vi "InstaCoverage Time Measurement - Copy.vi"(10 "test file paths":path[](array[path]), 11 "All Test":bool=TRUE) -> (2 "ICov Results":enum16{"PASSED", "FAILED", "ERROR"}[](array[ring]), 3 "ICov Testing time (seconds)":dbl)   [LabVIEW 2018]
uses:
  <vilib>/InstaCoverage/Pro/InstaCoverage_API/Run Tests From Project By Path.vi
  <vilib>/InstaCoverage/Core/TestSuite/TestSuite.lvclass
  <vilib>/InstaCoverage/Pro/InstaCoveragePro.lvlib
panel:
  out "Project Path":string
  # "If \"All Test\" is true, then all tests will be executed independelntly \nof \"test file paths\"."
  # "ICov"
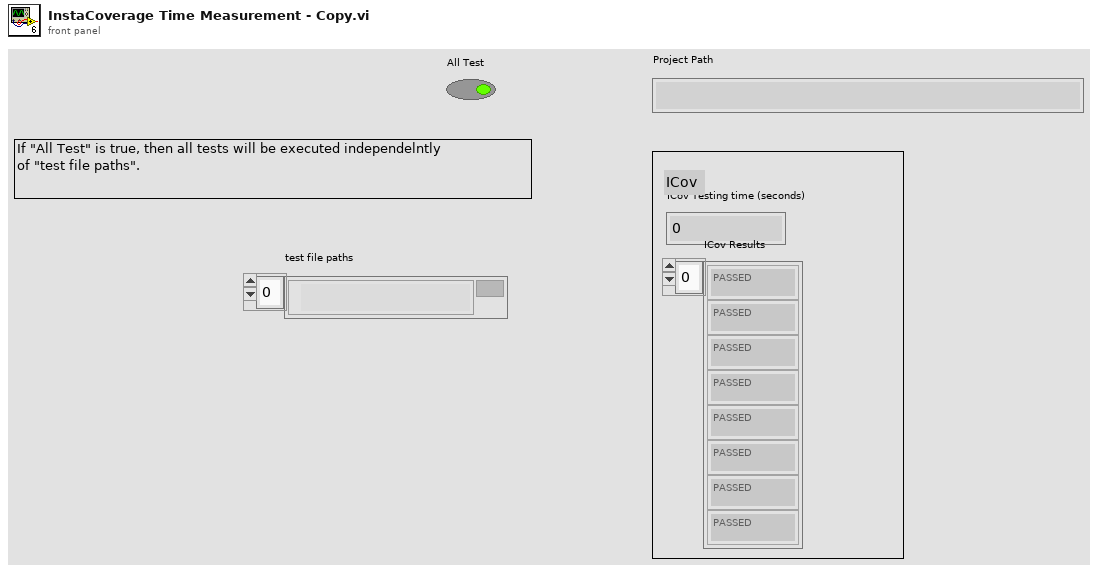
[diagram p1: front panel]
types:
  T1 = typedef "InstaCoverageCore.lvlib/APIResultEnum.ctl" = enum16{"PASSED", "FAILED", "ERROR", "NONE"}
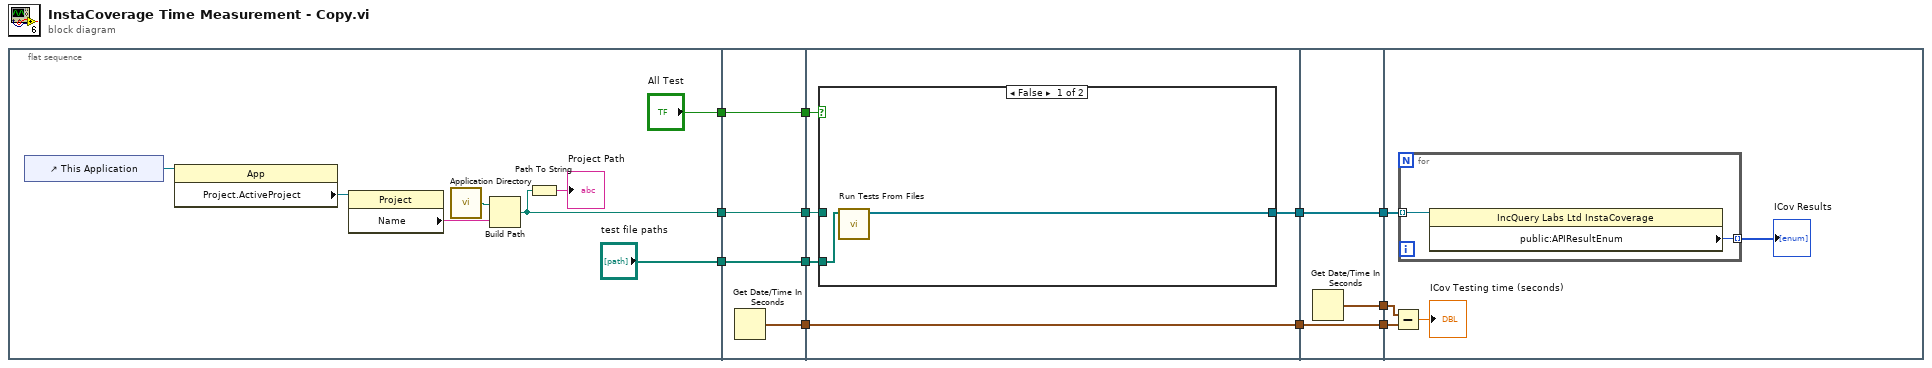
[diagram p0: block diagram]
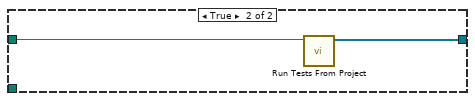
[diagram p2: hidden frame]
diagram:
  n1 = flat-sequence {
    tunnel: [w19] -> w5
    tunnel: ["All Test"] -> w3
    tunnel: ["test file paths"] -> w1
    tunnel: [w24] -> w9
    tunnel: [w23] -> w6
    tunnel: w5 -> [w23]
    tunnel: [w22] -> w4
    tunnel: w3 -> [w22]
    tunnel: [w21] -> w2
    tunnel: w1 -> [w21]
    tunnel: [w29] -> w10
    tunnel: w9 -> [w29]
    tunnel: [w27] -> w7
    tunnel: w6 -> [w28]
    tunnel: w4 -> [w26]
    tunnel: w2 -> [w25]
    tunnel: [w36] -> w12
    tunnel: [w35] -> w11
    tunnel: w10 -> [w35]
    tunnel: [w34] -> w8
    tunnel: w7 -> [w34]
    tunnel: w12 -> [w39]
    tunnel: w11 -> [w40]
    tunnel: w8 -> [w38]
    frame #0 {
      n2 = control-ref of="This Application"() -> (w14:refnum<vi>)
      n3 = property class="App"(reference=w14) -> ("Project.ActiveProject"=w15:refnum<vi>)  [unwired: 1 in, 2 out]
      n4 = property class="Project"(reference=w15) -> ("Name"=w13:string)  [unwired: 1 in, 2 out]
      n5 = call <vilib>:"Application Directory.vi"() -> ("Application Directory"=w18:path)
      n6 = Build Path(base path=w18, name or relative path=w13) -> (appended path=w19:path)
      n7 = Path To String(path=w19) -> (string=→"Project Path":string)
    }
    frame #1 {
      n8 = Get Date/Time In Seconds() -> (seconds since 1Jan1904=w24:timestamp)
    }
    frame #2 {
      n9 = case shown="False" w26 {
        tunnel: w28 -> [_ w33]
        tunnel: [w31 w32] -> w27
        tunnel: w25 -> [w30 _]
        frame False {
          n10 = call <vilib>:"Run Tests From Files.vi"("Path[] configs"=w30) -> ("TestSuite[] out"=w31:refnum<class "TestSuite.lvclass">[])  [unwired: 9 in, 1 out]
        }
        frame True {
          n11 = call-poly <vilib>:"Run Tests From Project.vi"("Path lvProject"=w33) -> ("TestSuite[] results"=w32:refnum<class "TestSuite.lvclass">[])  [unwired: 9 in, 1 out]
        }
      }
    }
    frame #3 {
      n12 = Get Date/Time In Seconds() -> (seconds since 1Jan1904=w36:timestamp)
    }
    frame #4 {
      n13 = Subtract(x=w39, y=w40) -> (x-y=→"ICov Testing time (seconds)":dbl)
      n14 = for {
        tunnel: w38 -> [w42] mode=indexing
        tunnel: [w43] -> w37 mode=indexing
        n15 = property class="IncQuery Labs Ltd InstaCoverage"(reference=w42) -> ("public:APIResultEnum"=w43:T1)  [unwired: 1 in, 2 out]
      }
      "ICov Results" <- w37
    }
  }
